vi "Close Holes.vi"(9 "Start Angle":dbl, 11 "Preliminary Arc Size":dbl) -> (1 "Final Arc Size":dbl, 3 "Final Angle":dbl)   [LabVIEW 2019, in "Zen Analytics.lvlib" / "Zen Analytics.lvclass"]
uses:
  Zen Analytics.lvclass
panel:
  out "error out":errorcluster
  in  "error in (no error)":errorcluster
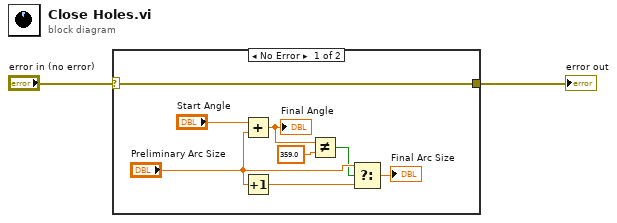
[diagram p0: block diagram]
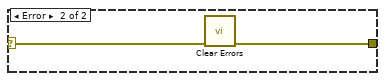
[diagram p2: hidden frame]
diagram:
  n1 = case shown="No Error" "error in (no error)" {
    selector: "error in (no error)" -> [w3 w12]
    tunnel: [w3 w11] -> w1
    frame No Error {
      n2 = Add(x="Start Angle", y="Preliminary Arc Size") -> (x+y=w8:dbl)
      "Final Angle" <- w8
      n3 = Increment(x="Preliminary Arc Size") -> (x+1=w9:dbl)
      n4 = Not Equal?(x=w8, y=359.0 ("x")) -> (x != y?=w6:bool)
      n5 = Select(t="Preliminary Arc Size", s=w6, f=w9) -> (s? t:f=→"Final Arc Size":dbl)
    }
    frame Error {
      n6 = call <vilib>:"Clear Errors.vi"("error in (no error)"=w12) -> ("error out"=w11:errorcluster)  [unwired: 5 in, 1 out]
    }
  }
  "error out" <- w1
